vi "BRig_RT__Case_Exp__State_CuePre__v3.vi"(0 "input_dataCurrent":u16[](array[numeric]), 1 "input_dataTrial":u16[][](array[numeric]), 3 "input_Cue2":bool, 6 "input_I_lick":bool, 7 "input_dataExp":u16[](array[numeric]), 9 "input_arrTrig":bool[](array[boolean])) -> (12 "output_state":T1, 13 "output_arrTrig":bool[](array[boolean]), 14 "output_dataCurrent":u16[](array[numeric]), 15 "output_dataTrial":u16[][](array[numeric]))   [LabVIEW 2014]
uses:
  myRIO_BRig_RT__Case_Exp_stateList.ctl
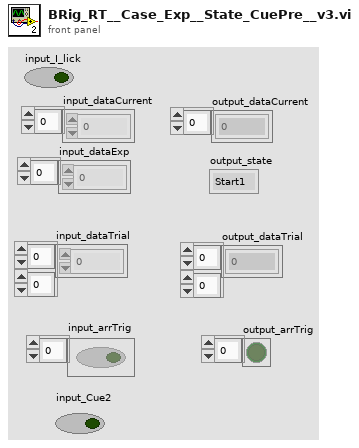
[diagram p1: front panel]
types:
  T1 = typedef "myRIO_BRig_RT__Case_Exp_stateList.ctl" = enum16{"Start1", "Start2", "Start3", "saveSettings1", "saveSettings2", "saveSettings3", "saveSettings4", "saveSettings_LC_ENL_l1", "saveSettings_LC_ENL_l2", "saveSettings_LC_Cue_l1", "saveSettings_LC_Cue_l2", "saveSettings6_LC_l1_Other", "SaveSettings6_LC_l2_Other", "setSettings_Audio", "setSettings_Laser", "initBlock_pre", "initBlock", "initBlock2", "initBlock_post", "initTrial_pre", "initTrial", "initTrial2", "initTrial3", "initTrial4", "initTrial_LC_ENL1", "initTrial_LC_Cue1", "initTrial_LC_Cue1_2", "initTrial_LC_Sel", "initTrial_post", "ENL1_pre", "ENL1", "ENL1_post", "ENL1Penalty_pre", "ENL1Penalty", "ENL2_pre", "ENL2", "ENL2Penalty_pre", "ENL2Penalty", "Cue1_pre", "Cue1", "Cue1_post", "Cue1Penalty_pre", "Cue1Penalty", "Cue2_pre", "Cue2", "Cue2Penalty_pre", "Cue2Penalty", "Selection_pre", "Selection", "Select_post", "SelectReward_pre", "SelectReward", "SelectRewardPost_pre", "SelectRewardPost", "SelectWrong_pre", "SelectWrong", "SelectWrong_post", "SelectTimeout_pre", "SelectTimeout", "SelectTimeout_post", "endTrial_pre", "endTrial1", "endTrial2", "endTrial3", "endTrial_post", "endBlock_pre", "endBlock", "endBlock_post", "endExp", "commConnect", "commUpload_pre", "commUpload_dataBlock", "commUpload_dataCurrent", "commUpload_dataExp", "commUpload_dataLC", "commUpload_dataTrial", "commUpload_post", "saveData_pre", "saveData_dataBlock", "saveData_dataCurrent", "saveData_dataExp", "saveData_dataLC", "saveData_dataTrial", "saveData_post", "empty_endBlock1", "empty_endBlock2", "empty_endTrial1", "empty_endTrial2", "empty_endTrial3", "empty_endTrial4", "empty_endTrial5", "dummyState", "dummyState_endBlock", "FreeReward_pre", "FreeReward", "FreeRewardPost_pre", "FreeRewardPost"}
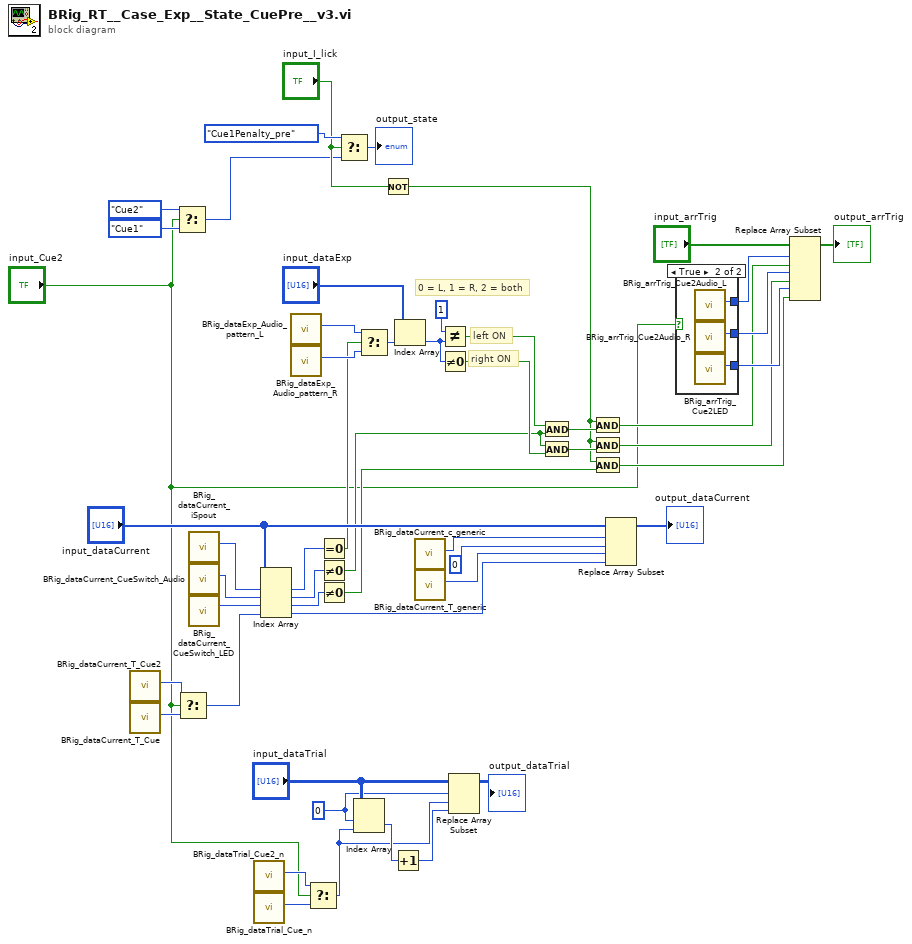
[diagram p0: block diagram]
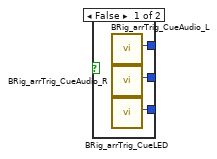
[diagram p2: hidden frame]
diagram:
  w11 = 0
  # "right ON"
  # "left ON"
  # "0 = L, 1 = R, 2 = both"
  n1 = call "BRig_dataCurrent_T_Cue2.vi"() -> ("output_T_Cue2"=w6:i32)  [unwired: 11 in]
  n2 = call "BRig_dataCurrent_T_Cue.vi"() -> ("output_T_Cue"=w7:i32)  [unwired: 11 in]
  n3 = Select(t=myRIO_BRig_RT__Case_Exp_stateList."Cue2", s="input_Cue2", f=myRIO_BRig_RT__Case_Exp_stateList."Cue1" ("Enum")) -> (s? t:f=w9:T1)
  n4 = Select(t=w6, s="input_Cue2", f=w7) -> (s? t:f=w5:i32)
  n5 = call "BRig_dataCurrent_iSpout.vi"() -> ("output_iSpout"=w33:i32)  [unwired: 11 in]
  n6 = call "BRig_dataCurrent_CueSwitch_Audio.vi"() -> ("output_CueSwitch_Audio"=w37:i32)  [unwired: 11 in]
  n7 = call "BRig_dataCurrent_CueSwitch_LED.vi"() -> ("output_CueSwitch_LED"=w38:i32)  [unwired: 11 in]
  n8 = call "BRig_dataTrial_Cue2_n.vi"() -> ("output_Cue2_n"=w3:i32)  [unwired: 11 in]
  n9 = call "BRig_dataTrial_Cue_n.vi"() -> ("output_Cue_n"=w4:i32)  [unwired: 11 in]
  n10 = Index Array(array="input_dataCurrent", index #1=w33, index #2=w37, index #3=w38, index #4=w5) -> (element #1=w32:u16, element #2=w36:u16, element #3=w35:u16, element #4=w39:u16)
  n11 = call "BRig_dataExp_Audio_pattern_L.vi"() -> ("output_Audio_sp__L"=w47:i32)  [unwired: 11 in]
  n12 = call "BRig_dataExp_Audio_pattern_R.vi"() -> ("output_Audio_sp__R"=w48:i32)  [unwired: 11 in]
  n13 = Select(t=w3, s="input_Cue2", f=w4) -> (s? t:f=w2:i32)
  n14 = Equal To 0?(x=w32) -> (x = 0?=w31:bool)
  n15 = Not Equal To 0?(x=w36) -> (x != 0?=w34:bool)
  n16 = Not Equal To 0?(x=w35) -> (x != 0?=w27:bool)
  n17 = Select(t=myRIO_BRig_RT__Case_Exp_stateList."Cue1Penalty_pre" ("Enum"), s="input_I_lick", f=w9) -> (s? t:f=→"output_state":T1)
  n18 = Index Array(array="input_dataTrial", index (row)=w11, index (col)=w2) -> (element=w22:u16)
  n19 = Select(t=w47, s=w31, f=w48) -> (s? t:f=w49:i32)
  n20 = Not(x="input_I_lick") -> (.not. x?=w26:bool)
  n21 = Increment(x=w22) -> (x+1=w21:u16)
  n22 = Index Array(array="input_dataExp", index=w49) -> (element=w24:u16)
  n23 = call "BRig_dataCurrent_c_generic.vi"() -> ("output_count_generic"=w42:i32)  [unwired: 11 in]
  n24 = call "BRig_dataCurrent_T_generic.vi"() -> ("output_T_generic"=w41:i32)  [unwired: 11 in]
  n25 = Not Equal?(x=u16 1 ("y"), y=w24) -> (x != y?=w45:bool)
  n26 = Not Equal To 0?(x=w24) -> (x != 0?=w44:bool)
  n27 = Replace Array Subset(array="input_dataTrial", new element=w21, index (row)=w11, index (col)=w2) -> (→"output_dataTrial":u16[][])
  n28 = And(x=w45, y=w34) -> (x .and. y?=w29:bool)
  n29 = And(x=w34, y=w44) -> (x .and. y?=w28:bool)
  n30 = And(x=w26, y=w29) -> (x .and. y?=w13:bool)
  n31 = And(x=w26, y=w28) -> (x .and. y?=w14:bool)
  n32 = And(x=w26, y=w27) -> (x .and. y?=w15:bool)
  n33 = Replace Array Subset(array="input_dataCurrent", new element #1=u16 0 ("new element/subarray"), index #1=w42, new element #2=w39, index #2=w41) -> (→"output_dataCurrent":u16[])
  n34 = case shown="True" "input_Cue2" {
    tunnel: [w55 w58] -> w18
    tunnel: [w54 w57] -> w17
    tunnel: [w53 w56] -> w16
    frame False {
      n35 = call "BRig_arrTrig_CueAudio_L.vi"() -> ("output_CueAudio_L"=w55:i32)  [unwired: 11 in]
      n36 = call "BRig_arrTrig_CueAudio_R.vi"() -> ("output_CueAudio_R"=w54:i32)  [unwired: 11 in]
      n37 = call "BRig_arrTrig_CueLED.vi"() -> ("output_CueLED"=w53:i32)  [unwired: 11 in]
    }
    frame True {
      n38 = call "BRig_arrTrig_Cue2Audio_L.vi"() -> ("output_Cue2Audio_L"=w58:i32)  [unwired: 11 in]
      n39 = call "BRig_arrTrig_Cue2Audio_R.vi"() -> ("output_Cue2Audio_R"=w57:i32)  [unwired: 11 in]
      n40 = call "BRig_arrTrig_Cue2LED.vi"() -> ("output_Cue2LED"=w56:i32)  [unwired: 11 in]
    }
  }
  n41 = Replace Array Subset(array="input_arrTrig", new element #1=w13, index #1=w18, new element #2=w14, index #2=w17, new element #3=w15, index #3=w16) -> (→"output_arrTrig":bool[])
